vi "CH_LM DFM Downoad File.vi"(0 "Meter Index":i32, 1 "File Name (\"\")":string, 3 "Destination (empty path)":path, 5 "error in (no error)":errorcluster, 7 "Timeout / ms (3000)":i32=3000, 9 "Lock Timeout / ms (1000)":i32=1000) -> (11 "Lock timed out":bool, 14 "Meter Index":i32, 19 "error out":errorcluster)   [LabVIEW 2012, in "CH_LM.lvlib"]
doc: "This VI downloads a file from the LabMax meter to a host storage device.\n\n<B>Details:</B>\nThe host interface will provide facility for transferring a trend data file in meter mass storage to the host computer via the host interface. \n\nThe model for the facility will be:\n1. set file name\n2. open file\n3. fetch data record(s)\n4. close file.\n\nOnly one file will be open at any time.\n\n<B>Attention:</B> Failing to follow the above order for file data access will raise error -200. The open/close state of a file will not persist across after a power off/on cycle. All files will be closed after a power off/on cycle."
uses:
  CH_LM.lvlib
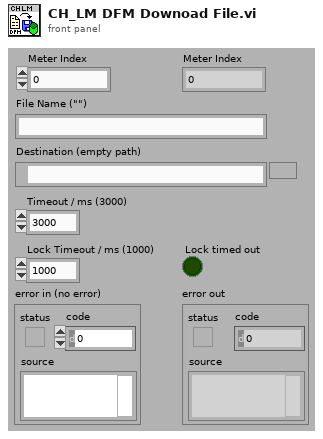
[diagram p1: front panel]
types:
  T1 = enum16{"open", "open or create", "create or replace", "create", "open (read only)"}
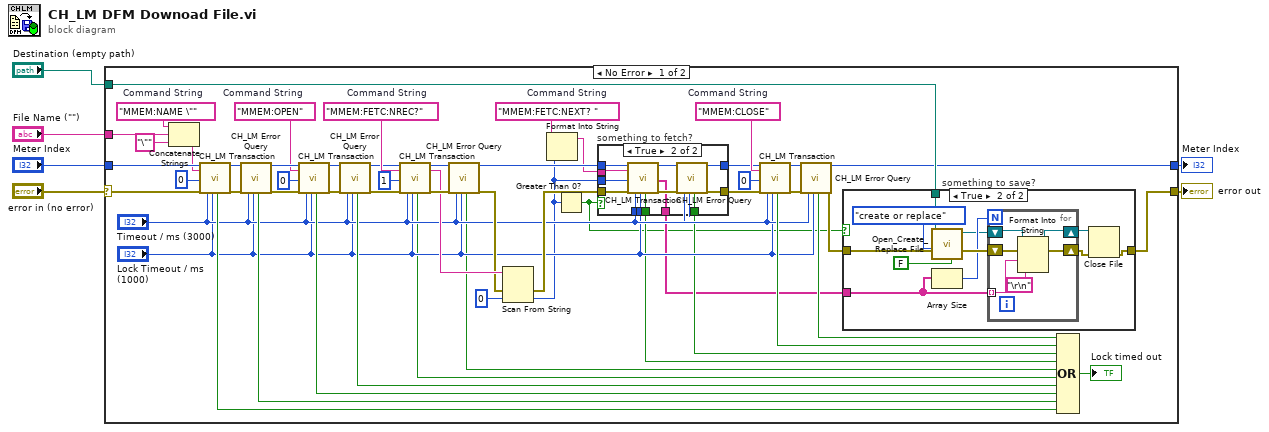
[diagram p0: block diagram]
diagram:
  n1 = case shown="No Error" "error in (no error)" {
    selector: "error in (no error)" -> [w60 w95]
    tunnel: [w11 w95] -> w6
    tunnel: "Meter Index" -> [w59 w94]
    tunnel: [w15 w94] -> w3
    tunnel: "File Name (\"\")" -> [w58 _]
    tunnel: "Destination (empty path)" -> [w17 _]
    frame No Error {
      w9 = "MMEM:FETC:NEXT? "  # Command String
      w28 = "MMEM:CLOSE"  # Command String
      w42 = "MMEM:FETC:NREC?"  # Command String
      w45 = "MMEM:OPEN"  # Command String
      w50 = "MMEM:NAME \""  # Command String
      n2 = Concatenate Strings(w50, w58, "\"" ("string")) -> (w52:string)
      n3 = call "CH_LM Transaction.vi"("Meter Index"=w59, "Command String"=w52, "NofStrings (-1:all)"=0 ("t"), "error in (no error)"=w60, "Timeout / ms (3000)"="Timeout / ms (3000)", "Lock Timeout / ms (1000)"="Lock Timeout / ms (1000)") -> ("Lock timed out"=w54:bool, "Meter Index"=w57:i32, "error out"=w56:errorcluster)  [unwired: 11 out]
      n4 = call "CH_LM Error Query.vi"("Meter Index"=w57, "error in (no error)"=w56, "Timeout / ms (3000)"="Timeout / ms (3000)", "Lock Timeout / ms (1000)"="Lock Timeout / ms (1000)") -> ("Lock timed out"=w55:bool, "Meter Index"=w47:i32, "error out"=w46:errorcluster)  [unwired: 13 out]
      n5 = call "CH_LM Transaction.vi"("Meter Index"=w47, "Command String"=w45, "NofStrings (-1:all)"=0, "error in (no error)"=w46, "Timeout / ms (3000)"="Timeout / ms (3000)", "Lock Timeout / ms (1000)"="Lock Timeout / ms (1000)") -> ("Lock timed out"=w44:bool, "Meter Index"=w48:i32, "error out"=w49:errorcluster)  [unwired: 11 out]
      n6 = call "CH_LM Error Query.vi"("Meter Index"=w48, "error in (no error)"=w49, "Timeout / ms (3000)"="Timeout / ms (3000)", "Lock Timeout / ms (1000)"="Lock Timeout / ms (1000)") -> ("Lock timed out"=w43:bool, "Meter Index"=w39:i32, "error out"=w38:errorcluster)  [unwired: 13 out]
      n7 = call "CH_LM Transaction.vi"("Meter Index"=w39, "Command String"=w42, "NofStrings (-1:all)"=1, "error in (no error)"=w38, "Timeout / ms (3000)"="Timeout / ms (3000)", "Lock Timeout / ms (1000)"="Lock Timeout / ms (1000)") -> ("Lock timed out"=w21:bool, "Meter Index"=w41:i32, "Response"=w34:string, "error out"=w40:errorcluster)  [unwired: 10 out]
      n8 = call "CH_LM Error Query.vi"("Meter Index"=w41, "error in (no error)"=w40, "Timeout / ms (3000)"="Timeout / ms (3000)", "Lock Timeout / ms (1000)"="Lock Timeout / ms (1000)") -> ("Lock timed out"=w20:bool, "Meter Index"=w27:i32, "error out"=w32:errorcluster)  [unwired: 13 out]
      n9 = Scan From String(input string=w34, error in=w32, default 1=0 ("default value 1")) -> (error out=w26:errorcluster, output 1=w10:i32)  [unwired: 2 in, 2 out]
      n10 = Format Into String(initial string=w9, w10) -> (resulting string=w8:string)  [unwired: 2 in, 1 out]
      n11 = Greater Than 0?(x=w10) -> (x > 0?=w7:bool)
      n12 = case "something to fetch?" shown="True" w7 {
        tunnel: w8 -> [_ w91]
        tunnel: w27 -> [w80 w90]
        tunnel: w26 -> [w79 w89]
        tunnel: "Timeout / ms (3000)" -> [_ w88]
        tunnel: "Lock Timeout / ms (1000)" -> [_ w87]
        tunnel: [_ w86] -> w19
        tunnel: [_ w85] -> w18
        tunnel: w10 -> [_ w84]
        tunnel: [w79 w83] -> w14
        tunnel: [w80 w82] -> w13
        tunnel: [_ w81] -> w12
        frame False {
        }
        frame True {
          n13 = call "CH_LM Transaction.vi"("Meter Index"=w90, "Command String"=w91, "NofStrings (-1:all)"=w84, "error in (no error)"=w89, "Timeout / ms (3000)"=w88, "Lock Timeout / ms (1000)"=w87) -> ("Lock timed out"=w86:bool, "Meter Index"=w92:i32, "Response Array"=w81:string[], "error out"=w93:errorcluster)  [unwired: 10 out]
          n14 = call "CH_LM Error Query.vi"("Meter Index"=w92, "error in (no error)"=w93, "Timeout / ms (3000)"=w88, "Lock Timeout / ms (1000)"=w87) -> ("Lock timed out"=w85:bool, "Meter Index"=w82:i32, "error out"=w83:errorcluster)  [unwired: 13 out]
        }
      }
      n15 = call "CH_LM Transaction.vi"("Meter Index"=w13, "Command String"=w28, "NofStrings (-1:all)"=0, "error in (no error)"=w14, "Timeout / ms (3000)"="Timeout / ms (3000)", "Lock Timeout / ms (1000)"="Lock Timeout / ms (1000)") -> ("Lock timed out"=w24:bool, "Meter Index"=w30:i32, "error out"=w29:errorcluster)  [unwired: 11 out]
      n16 = call "CH_LM Error Query.vi"("Meter Index"=w30, "error in (no error)"=w29, "Timeout / ms (3000)"="Timeout / ms (3000)", "Lock Timeout / ms (1000)"="Lock Timeout / ms (1000)") -> ("Lock timed out"=w25:bool, "Meter Index"=w15:i32, "error out"=w16:errorcluster)  [unwired: 13 out]
      n17 = case "something to save?" shown="True" w7 {
        tunnel: w17 -> [_ w72]
        tunnel: w16 -> [w61 w71]
        tunnel: w12 -> [_ w66]
        tunnel: [w61 w65] -> w11
        frame False {
        }
        frame True {
          n18 = call <vilib>:"Open_Create_Replace File.vi"("advisory dialog? (display:T)"=FALSE, "error in (no error)"=w71, "function (open:0)"=T1."create or replace", "file path"=w72) -> ("error out"=w69:errorcluster, "refnum"=w64:refnum<file>)  [unwired: 3 in, 3 out]
          n19 = Array Size(array=w66) -> (size(s)=w67:i32)
          n20 = for {
            N: w67 -> [_]
            shift-right: [w75] -> w68
            shift-left: w69 -> [w76]
            tunnel: w66 -> [w74] mode=indexing
            shift-right: [w77] -> w70
            shift-left: w64 -> [w78]
            n21 = Format Into String(initial string=w78, error in=w76, w74, "\r\n") -> (resulting string=w77:refnum<file>, error out=w75:errorcluster)  [unwired: 1 in]
          }
          n22 = Close File(refnum=w70, error in=w68) -> (error out=w65:errorcluster)  [unwired: 1 out]
        }
      }
      n23 = Compound Arithmetic op=OR(w25, w24, w18, w19, w20, w21, w43, w44, w55, w54) -> (→"Lock timed out":bool)
    }
    frame Error {
    }
  }
  "error out" <- w6
  "Meter Index" <- w3
